vi "RoboTaxi_mainVI.vi"() -> ()   [LabVIEW 2022 SP3]
doc: "Demonstrates how to open a connection to an TCP server, read the data being sent, and display the data on a chart. This VI is designed to stop if the TCP connection is terminated."
panel:
  in  "Interactive Mode 2":bool
  in  "Stop 2":bool
  in  "Path":path=path "C:/Users/rafae/Documents/My Files/UC Berkeley/Academics/Spring/ME 235 Microproc MS Des/Final Project/RoboTaxi/Lidar/PyLidar_class.py1.jpg"
  out "LiDAR Clustered Point Clouds":picture
  in  "Track 2":bool
  in  "Track 1":bool
  in  "Stop":bool
  in  "Server Closed":string="The server VI closed the connection."
  in  "IP Address":string="192.168.4.1"
  out "Response":string
  in  "Interactive Mode":bool
  in  "Stop Driving":bool
  in  "Right":bool
  in  "Left":bool
  in  "Backward":bool
  in  "Forward":bool
  # "Track Selection"
  # "Interactive Mode"
  # "(Real-Time Obstacle Avoidance)"
  # "Track 1"
  # "Track 2"
  # "Manual Control"
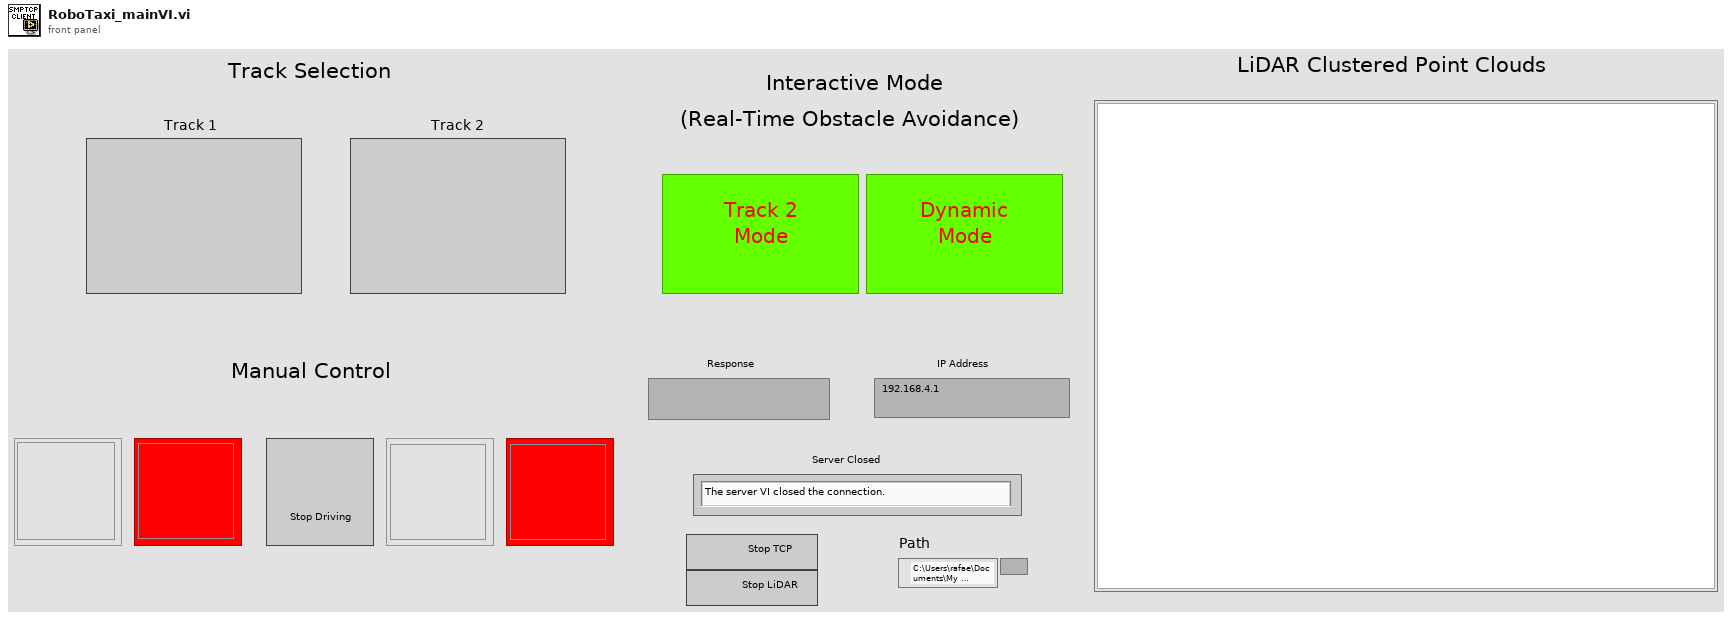
[diagram p1: front panel]
types:
  T1 = typedef "imagedata.ctl" = cluster{"image type":i32, "image depth":i32, "image":u8[], "mask":u8[], "colors":u32[], "Rectangle":cluster{"left":i16, "top":i16, "right":i16, "bottom":i16}}
  T2 = enum16{"Standard", "Buffered", "CRLF", "Immediate"}
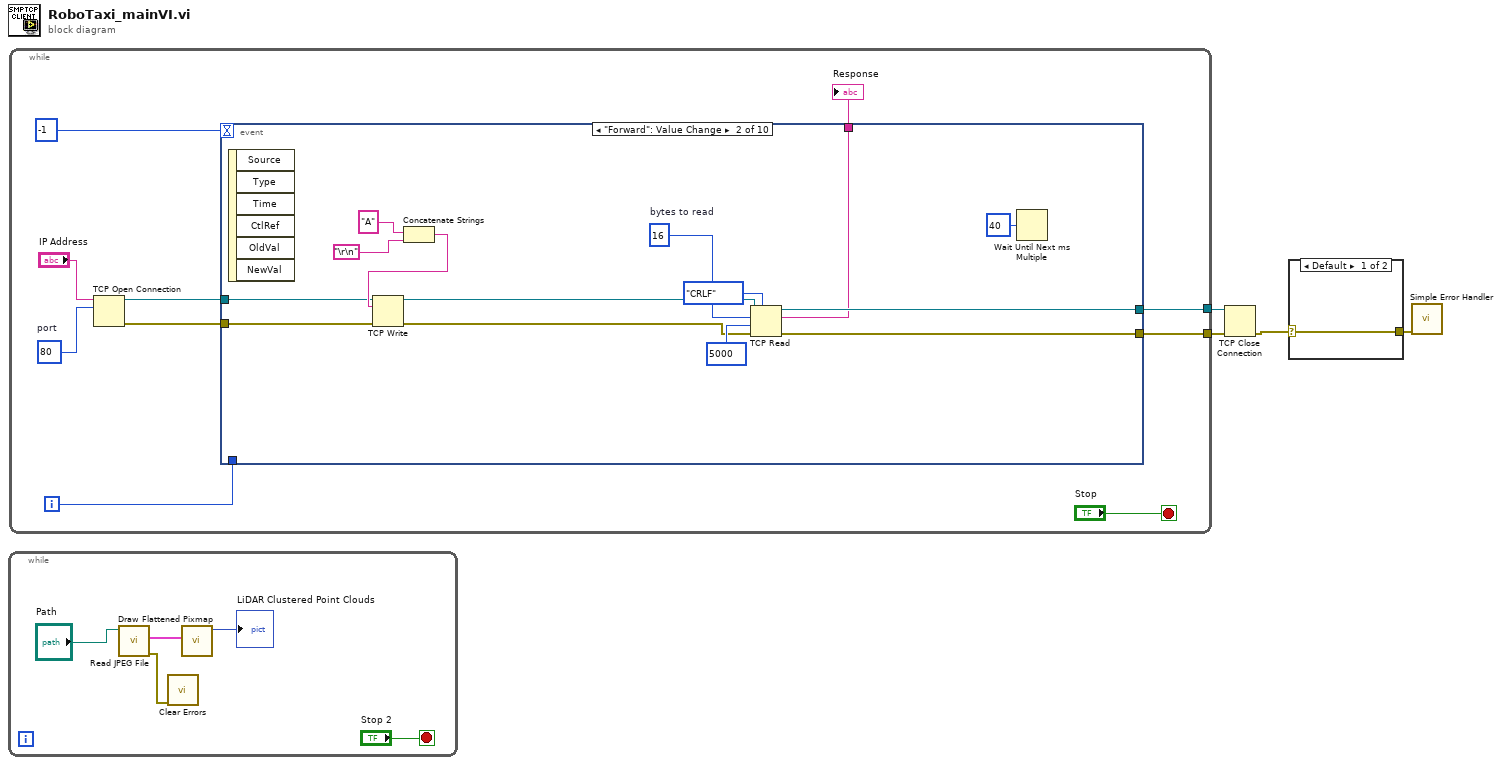
[diagram p0: block diagram]
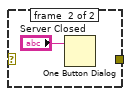
[diagram p2: hidden frame]
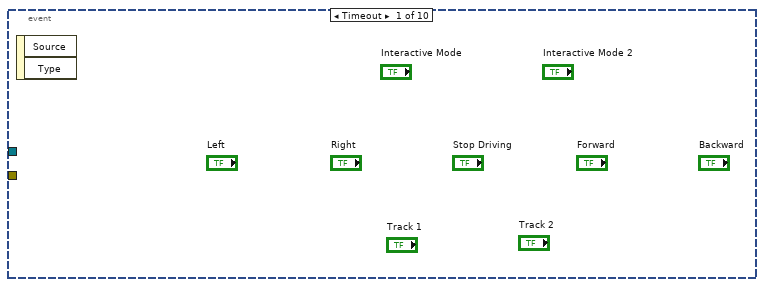
[diagram p3: hidden frame]
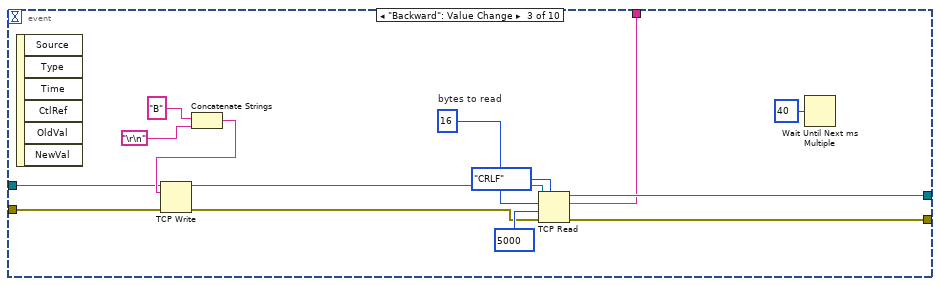
[diagram p4: hidden frame]
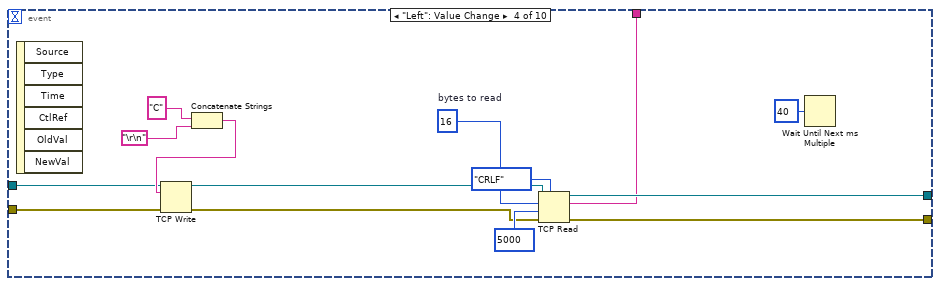
[diagram p5: hidden frame]
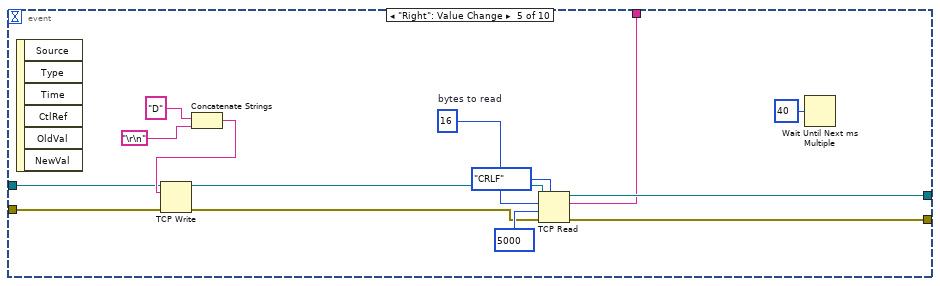
[diagram p6: hidden frame]
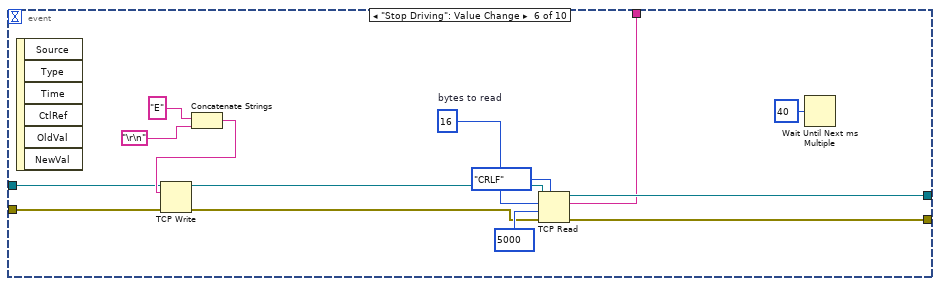
[diagram p7: hidden frame]
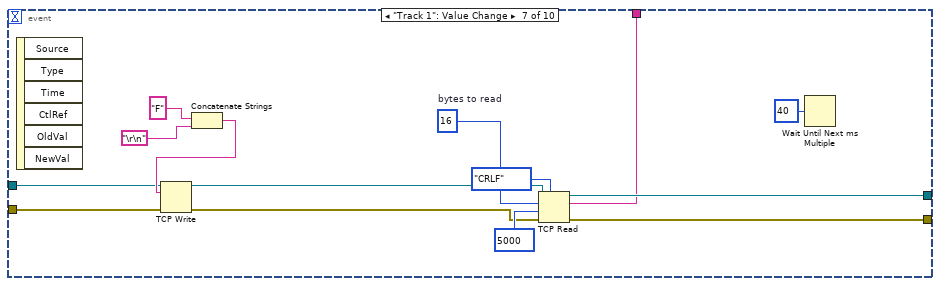
[diagram p8: hidden frame]
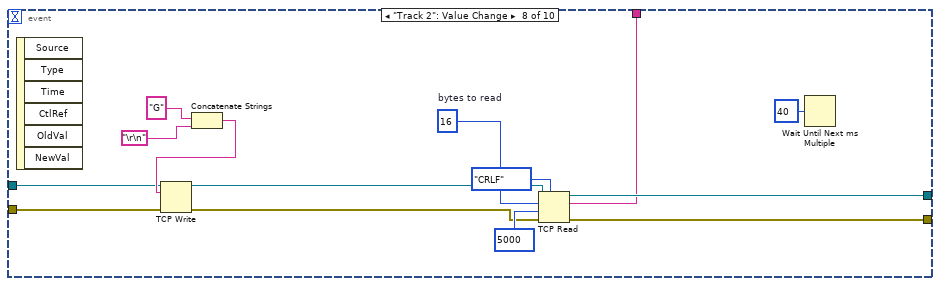
[diagram p9: hidden frame]
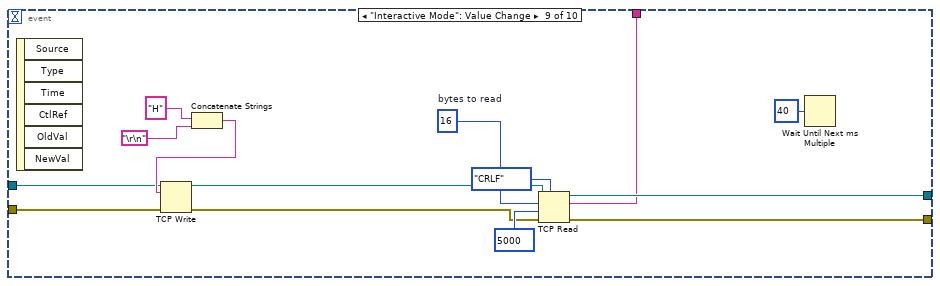
[diagram p10: hidden frame]
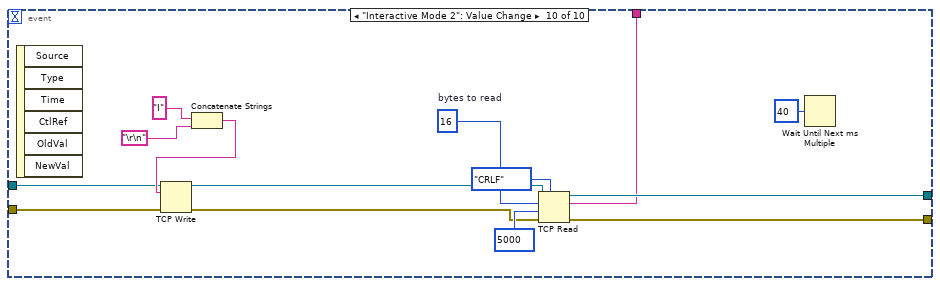
[diagram p11: hidden frame]
diagram:
  n1 = while {
    stop <- "Stop 2" stop-if-true
    n2 = call <vilib>:"Read JPEG File.vi"("path to JPEG file"="Path") -> ("error out"=w5:errorcluster, "image data"=w7:T1)  [unwired: 1 in, 8 out]
    n3 = call <vilib>:"Clear Errors.vi"("error in (no error)"=w5) -> ()  [unwired: 5 in, 2 out]
    n4 = call <vilib>:"Draw Flattened Pixmap.vi"("image data"=w7) -> ("new picture"=→"LiDAR Clustered Point Clouds":picture)  [unwired: 1 in, 7 out]
  }
  n5 = while {
    tunnel: [w13] -> w2
    tunnel: [w12] -> w1
    i -> [w18]
    stop <- "Stop" stop-if-true
    w16 = u16 80  # port
    n6 = TCP Open Connection(address="IP Address", remote port or service name=w16) -> (connection ID=w14:refnum<k5>, error out=w15:errorcluster)  [unwired: 3 in]
    n7 = event shown="[1] \"Forward\": Value Change" {
      selector: _ -> [_ _ _ _ _ _ _ _ _ _]
      dyn-events: _ -> [_ _ _ _ _ _ _ _ _ _]
      timeout: -1 -> [_ _ _ _ _ _ _ _ _ _]
      tunnel: w18 -> [_ _ _ _ _ _ _ _ _ _]
      tunnel: w15 -> [_ w24 w38 w52 w66 w80 w94 w108 w122 w136]
      tunnel: w14 -> [_ w23 w37 w51 w65 w79 w93 w107 w121 w135]
      tunnel: [_ w22 w36 w50 w64 w78 w92 w106 w120 w134] -> w13
      tunnel: [_ w21 w35 w49 w63 w77 w91 w105 w119 w133] -> w12
      tunnel: [_ w20 w34 w48 w62 w76 w90 w104 w118 w132] -> w11
      event Timeout {
        n8 = event-data() -> ()  [unwired: 1 in, 2 out]
      }
      event "Forward": Value Change {
        w33 = 16  # bytes to read
        n9 = event-data() -> ()  [unwired: 1 in, 6 out]
        n10 = Concatenate Strings("A" ("data in"), "\r\n") -> (w26:string)
        n11 = TCP Write(connection ID=w23, data in=w26, error in (no error)=w24) -> (connection ID out=w31:refnum<k5>, error out=w25:errorcluster)  [unwired: 1 in, 1 out]
        n12 = TCP Read(connection ID=w31, bytes to read=w33, error in (no error)=w25, 7:T2."CRLF" ("mode (standard)"), 9:5000 ("timeout ms (25000)")) -> (connection ID out=w21:refnum<k5>, data out=w20:string, error out=w22:errorcluster)
        n13 = Wait Until Next ms Multiple(millisecond multiple=u32 40) -> ()  [unwired: 1 out]
      }
      event "Backward": Value Change {
        w47 = 16  # bytes to read
        n14 = event-data() -> ()  [unwired: 1 in, 6 out]
        n15 = Concatenate Strings("B" ("data in"), "\r\n") -> (w40:string)
        n16 = TCP Write(connection ID=w37, data in=w40, error in (no error)=w38) -> (connection ID out=w45:refnum<k5>, error out=w39:errorcluster)  [unwired: 1 in, 1 out]
        n17 = TCP Read(connection ID=w45, bytes to read=w47, error in (no error)=w39, 7:T2."CRLF" ("mode (standard)"), 9:5000 ("timeout ms (25000)")) -> (connection ID out=w35:refnum<k5>, data out=w34:string, error out=w36:errorcluster)
        n18 = Wait Until Next ms Multiple(millisecond multiple=u32 40) -> ()  [unwired: 1 out]
      }
      event "Left": Value Change {
        w61 = 16  # bytes to read
        n19 = event-data() -> ()  [unwired: 1 in, 6 out]
        n20 = Concatenate Strings("C" ("data in"), "\r\n") -> (w54:string)
        n21 = TCP Write(connection ID=w51, data in=w54, error in (no error)=w52) -> (connection ID out=w59:refnum<k5>, error out=w53:errorcluster)  [unwired: 1 in, 1 out]
        n22 = TCP Read(connection ID=w59, bytes to read=w61, error in (no error)=w53, 7:T2."CRLF" ("mode (standard)"), 9:5000 ("timeout ms (25000)")) -> (connection ID out=w49:refnum<k5>, data out=w48:string, error out=w50:errorcluster)
        n23 = Wait Until Next ms Multiple(millisecond multiple=u32 40) -> ()  [unwired: 1 out]
      }
      event "Right": Value Change {
        w75 = 16  # bytes to read
        n24 = event-data() -> ()  [unwired: 1 in, 6 out]
        n25 = Concatenate Strings("D" ("data in"), "\r\n") -> (w68:string)
        n26 = TCP Write(connection ID=w65, data in=w68, error in (no error)=w66) -> (connection ID out=w73:refnum<k5>, error out=w67:errorcluster)  [unwired: 1 in, 1 out]
        n27 = TCP Read(connection ID=w73, bytes to read=w75, error in (no error)=w67, 7:T2."CRLF" ("mode (standard)"), 9:5000 ("timeout ms (25000)")) -> (connection ID out=w63:refnum<k5>, data out=w62:string, error out=w64:errorcluster)
        n28 = Wait Until Next ms Multiple(millisecond multiple=u32 40) -> ()  [unwired: 1 out]
      }
      event "Stop Driving": Value Change {
        w89 = 16  # bytes to read
        n29 = event-data() -> ()  [unwired: 1 in, 6 out]
        n30 = Concatenate Strings("E" ("data in"), "\r\n") -> (w82:string)
        n31 = TCP Write(connection ID=w79, data in=w82, error in (no error)=w80) -> (connection ID out=w87:refnum<k5>, error out=w81:errorcluster)  [unwired: 1 in, 1 out]
        n32 = TCP Read(connection ID=w87, bytes to read=w89, error in (no error)=w81, 7:T2."CRLF" ("mode (standard)"), 9:5000 ("timeout ms (25000)")) -> (connection ID out=w77:refnum<k5>, data out=w76:string, error out=w78:errorcluster)
        n33 = Wait Until Next ms Multiple(millisecond multiple=u32 40) -> ()  [unwired: 1 out]
      }
      event "Track 1": Value Change {
        w103 = 16  # bytes to read
        n34 = event-data() -> ()  [unwired: 1 in, 6 out]
        n35 = Concatenate Strings("F" ("data in"), "\r\n") -> (w96:string)
        n36 = TCP Write(connection ID=w93, data in=w96, error in (no error)=w94) -> (connection ID out=w101:refnum<k5>, error out=w95:errorcluster)  [unwired: 1 in, 1 out]
        n37 = TCP Read(connection ID=w101, bytes to read=w103, error in (no error)=w95, 7:T2."CRLF" ("mode (standard)"), 9:5000 ("timeout ms (25000)")) -> (connection ID out=w91:refnum<k5>, data out=w90:string, error out=w92:errorcluster)
        n38 = Wait Until Next ms Multiple(millisecond multiple=u32 40) -> ()  [unwired: 1 out]
      }
      event "Track 2": Value Change {
        w117 = 16  # bytes to read
        n39 = event-data() -> ()  [unwired: 1 in, 6 out]
        n40 = Concatenate Strings("G" ("data in"), "\r\n") -> (w110:string)
        n41 = TCP Write(connection ID=w107, data in=w110, error in (no error)=w108) -> (connection ID out=w115:refnum<k5>, error out=w109:errorcluster)  [unwired: 1 in, 1 out]
        n42 = TCP Read(connection ID=w115, bytes to read=w117, error in (no error)=w109, 7:T2."CRLF" ("mode (standard)"), 9:5000 ("timeout ms (25000)")) -> (connection ID out=w105:refnum<k5>, data out=w104:string, error out=w106:errorcluster)
        n43 = Wait Until Next ms Multiple(millisecond multiple=u32 40) -> ()  [unwired: 1 out]
      }
      event "Interactive Mode": Value Change {
        w131 = 16  # bytes to read
        n44 = event-data() -> ()  [unwired: 1 in, 6 out]
        n45 = Concatenate Strings("H" ("data in"), "\r\n") -> (w124:string)
        n46 = TCP Write(connection ID=w121, data in=w124, error in (no error)=w122) -> (connection ID out=w129:refnum<k5>, error out=w123:errorcluster)  [unwired: 1 in, 1 out]
        n47 = TCP Read(connection ID=w129, bytes to read=w131, error in (no error)=w123, 7:T2."CRLF" ("mode (standard)"), 9:5000 ("timeout ms (25000)")) -> (connection ID out=w119:refnum<k5>, data out=w118:string, error out=w120:errorcluster)
        n48 = Wait Until Next ms Multiple(millisecond multiple=u32 40) -> ()  [unwired: 1 out]
      }
      event "Interactive Mode 2": Value Change {
        w145 = 16  # bytes to read
        n49 = event-data() -> ()  [unwired: 1 in, 6 out]
        n50 = Concatenate Strings("I" ("data in"), "\r\n") -> (w138:string)
        n51 = TCP Write(connection ID=w135, data in=w138, error in (no error)=w136) -> (connection ID out=w143:refnum<k5>, error out=w137:errorcluster)  [unwired: 1 in, 1 out]
        n52 = TCP Read(connection ID=w143, bytes to read=w145, error in (no error)=w137, 7:T2."CRLF" ("mode (standard)"), 9:5000 ("timeout ms (25000)")) -> (connection ID out=w133:refnum<k5>, data out=w132:string, error out=w134:errorcluster)
        n53 = Wait Until Next ms Multiple(millisecond multiple=u32 40) -> ()  [unwired: 1 out]
      }
    }
    "Response" <- w11
  }
  n54 = TCP Close Connection(connection ID=w1, error in (no error)=w2) -> (error out=w3:errorcluster)  [unwired: 1 in, 1 out]
  n55 = case shown="Default" w3 {
    selector: w3 -> [w146 _]
    tunnel: [w146 _] -> w4
    frame #0 {
    }
    frame #1 {
      n56 = One Button Dialog(message="Server Closed") -> ()  [unwired: 1 in, 1 out]
    }
  }
  n57 = call <vilib>:"Simple Error Handler.vi"("error in (no error)"=w4) -> ()  [unwired: 4 in, 5 out]
